vi "laser_control of Tank 2.vi"() -> ()   [LabVIEW 2012]
panel:
  out "i":dbl
  in  "Boolean":bool
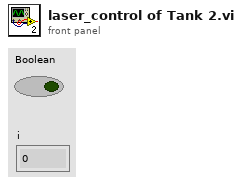
[diagram p1: front panel]
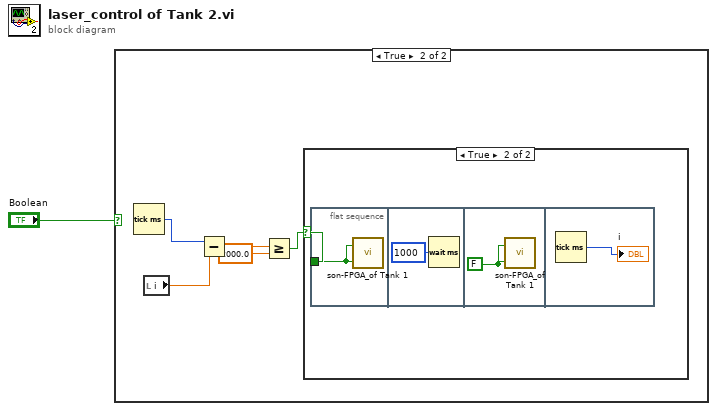
[diagram p0: block diagram]
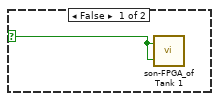
[diagram p3: hidden frame]
diagram:
  n1 = case shown="True" "Boolean" {
    frame False {
    }
    frame True {
      n2 = Tick Count (ms)() -> (millisecond timer value=w5:u32)
      n3 = local read "i"() -> (w6:dbl)
      n4 = Subtract(x=w5, y=w6) -> (x-y=w4:dbl)
      n5 = Greater Or Equal?(x=w4, y=2000.0) -> (x >= y?=w2:bool)
      n6 = case shown="True" w2 {
        selector: w2 -> [w7 w8]
        frame False {
          n7 = call "son-FPGA_of Tank 1.vi"("Port9/DIO8"=w7, "stop"=w7) -> ()  [unwired: 1 in]
        }
        frame True {
          n8 = flat-sequence {
            tunnel: w8 -> [w9]
            frame #0 {
              n9 = call "son-FPGA_of Tank 1.vi"("Port9/DIO8"=w9, "stop"=w9) -> ()  [unwired: 1 in]
            }
            frame #1 {
              n10 = Wait (ms)(milliseconds to wait=u32 1000) -> ()  [unwired: 1 out]
            }
            frame #2 {
              w11 = FALSE ("Port9/DIO8")
              n11 = call "son-FPGA_of Tank 1.vi"("Port9/DIO8"=w11, "stop"=w11) -> ()  [unwired: 1 in]
            }
            frame #3 {
              n12 = Tick Count (ms)() -> (millisecond timer value=→"i":u32)
            }
          }
        }
      }
    }
  }
